vi "Abort Session.vi"(8 "error in (no error)":errorcluster, 11 "SLSC Local in":refnum<class "SLSC Local.lvclass">) -> (0 "error out":errorcluster, 3 "SLSC Local out":refnum<class "SLSC Local.lvclass">)   [LabVIEW 2015, in "SLSC Local.lvclass"]
uses:
  SLSC Local.lvclass
  <vilib>/SLSC/SLSC.lvlib
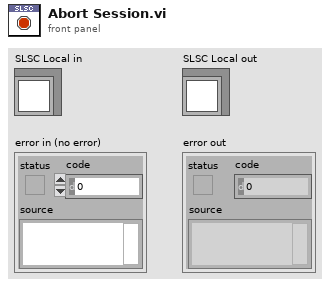
[diagram p1: front panel]
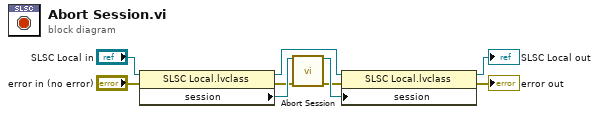
[diagram p0: block diagram]
diagram:
  n1 = property class="SLSC Local.lvclass"(reference="SLSC Local in", error in="error in (no error)") -> (reference out=w7:refnum<class "SLSC Local.lvclass">, error out=w3:errorcluster, "session"=w6:refnum<k21>)
  n2 = call <vilib>:"Abort Session.vi"("session in"=w6, "error in (no error)"=w3) -> ("session out"=w5:refnum<k21>, "error out"=w2:errorcluster)  [unwired: 12 in]
  n3 = property class="SLSC Local.lvclass"(reference=w7, error in=w2, "session"=w5) -> (reference out=→"SLSC Local out":refnum<class "SLSC Local.lvclass">, error out=→"error out":errorcluster)
